vi "UI - Initiate Connection.vi"(8 "error in (no error)":errorcluster, 10 "Controller Address":string, 11 "Message Queue":refnum<queue>) -> (0 "error out":errorcluster, 1 "Connected?":bool, 3 "dup Message Queue":refnum<queue>)   [LabVIEW 2017]
uses:
  Support/Message Queue/Message Cluster.ctl
  Controls/Manual Control.ctl
  Controls/Variable References.ctl
  Globals/Host/Global - Configuration Options.vi
  Globals/Host/Global - UI Streams and Variables.vi
  Support/Message Queue/Message Queue.lvlib
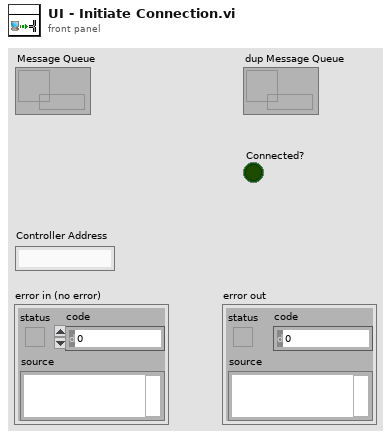
[diagram p1: front panel]
types:
  T1 = typedef "Manual Control.ctl" = cluster{"Actuator Settings":cluster{"Actuator Name":string, "Unpowered State":i16, "Output Port":u32, "Emergency State":i16, "Blank Button":bool, "Open Time [ms]":i16, "Close Time [ms]":i16}[]}
  T2 = typedef "Message Queue.lvlib/Message Cluster.ctl" = cluster{"Message":string, "Message Data":variant}
  T3 = typedef "Variable References.ctl" = cluster{"CPU Usage":refnum<k21>, "Buffer Backlog":refnum<k21>, "Contiguous Memory":refnum<k21>, "Drive Space":refnum<k21>, "Actual Loop Period":refnum<k21>, "LC Data":refnum<k21>, "PS Data":refnum<k21>, "TC Data":refnum<k21>, "Valve States":refnum<k21>, "AC Timer":refnum<k21>}
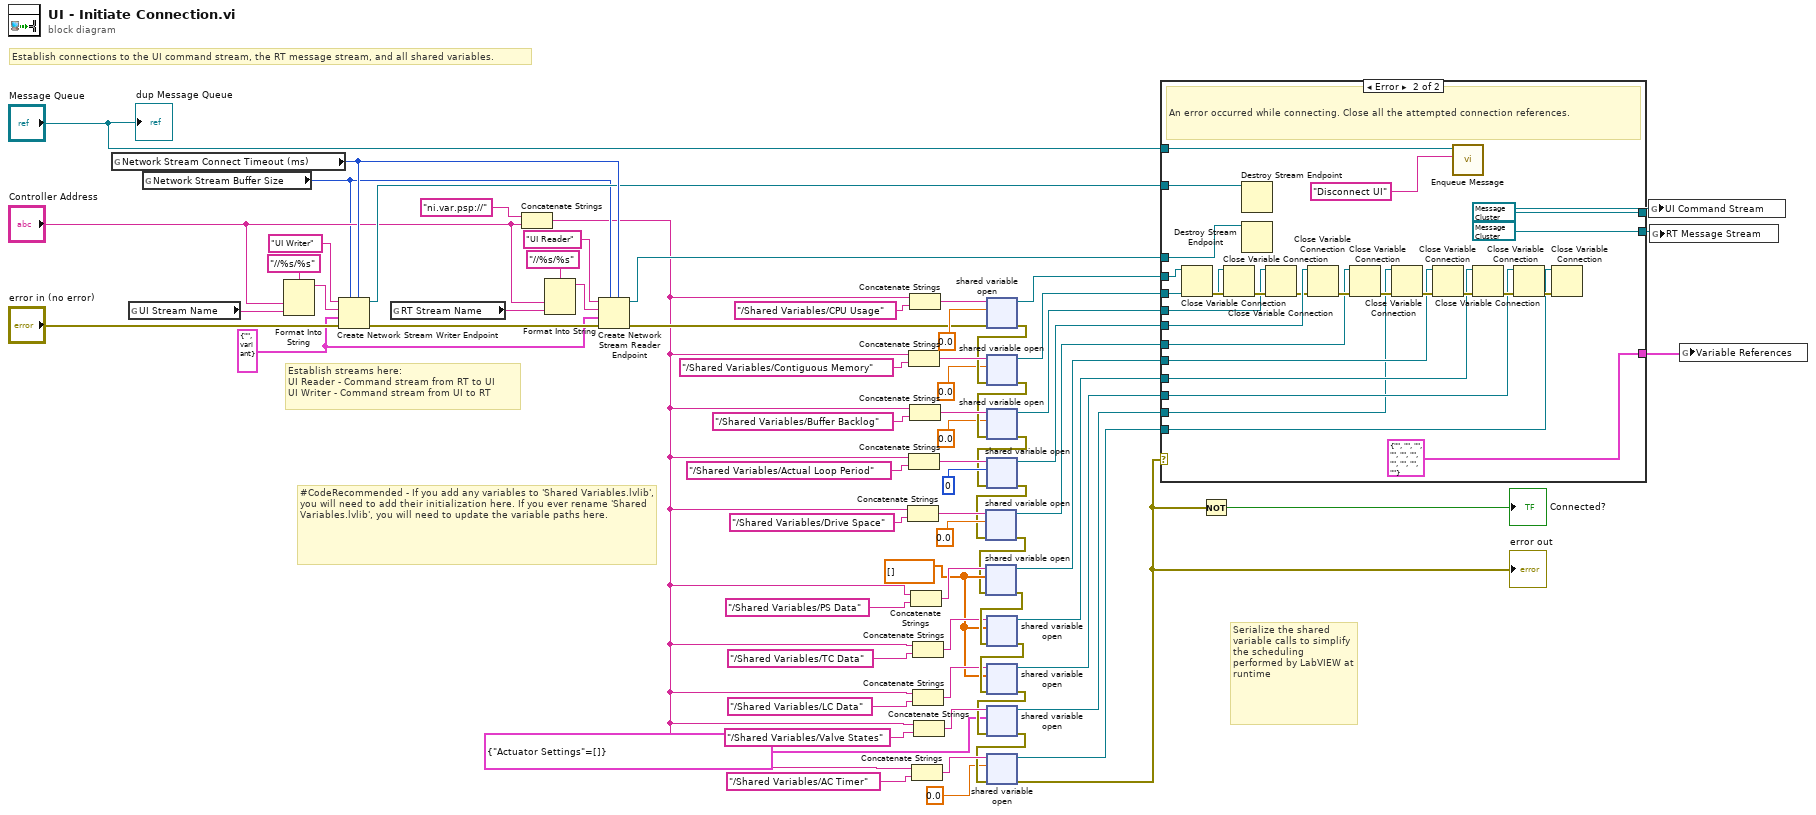
[diagram p0: block diagram]
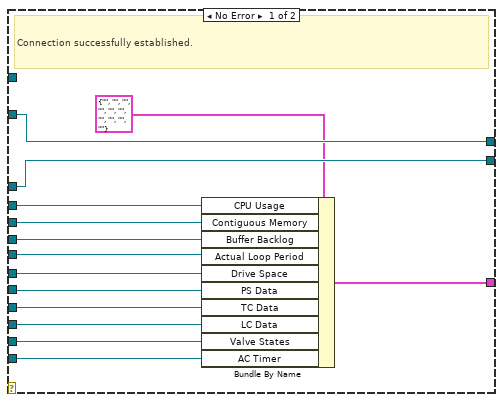
[diagram p2: hidden frame]
diagram:
  w20 = dbl[] []
  w29 = T2 {"Message"="", "Message Data"=variant} ("Message Cluster")
  # "Establish connections to the UI command stream, the RT message stream, and all shared variables."
  # "#CodeRecommended - If you add any variables to 'Shared Variables.lvlib', you will need to add their initialization here. If you ever rename 'Shared Variables.lvlib', you will need to update the variable paths here."
  # "Establish streams here:\nUI Reader - Command stream from RT to UI\nUI Writer - Command stream from UI to RT"
  # "Serialize the shared variable calls to simplify the scheduling performed by LabVIEW at runtime"
  n1 = global read "Global - Configuration Options.vi" "Network Stream Connect Timeout (ms)"() -> (w61:i32)
  n2 = global read "Global - Configuration Options.vi" "UI Stream Name"() -> (w67:string)
  n3 = global read "Global - Configuration Options.vi" "Network Stream Buffer Size"() -> (w31:i32)
  n4 = Format Into String(format string="//%s/%s", "Controller Address", w67) -> (resulting string=w66:string)  [unwired: 2 in, 1 out]
  n5 = Create Network Stream Writer Endpoint(5:w61, 7:w31, 8:"error in (no error)", 9:w29, 10:w66, 11:"UI Writer" ("reader name")) -> (0:w62:errorcluster, 3:w41:refnum<k21>)  [unwired: 1 in]
  n6 = global read "Global - Configuration Options.vi" "RT Stream Name"() -> (w70:string)
  n7 = Concatenate Strings("ni.var.psp://", "Controller Address") -> (w9:string)
  n8 = Format Into String(format string="//%s/%s", "Controller Address", w70) -> (resulting string=w69:string)  [unwired: 2 in, 1 out]
  n9 = Create Network Stream Reader Endpoint(5:w61, 7:w31, 8:w62, 9:w29, 10:w69, 11:"UI Reader" ("writer name")) -> (0:w58:errorcluster, 3:w42:refnum<k21>)  [unwired: 1 in]
  n10 = Concatenate Strings(w9, "/Shared Variables/Drive Space") -> (w36:string)
  n11 = Concatenate Strings(w9, "/Shared Variables/Contiguous Memory") -> (w54:string)
  n12 = Concatenate Strings(w9, "/Shared Variables/Actual Loop Period") -> (w50:string)
  n13 = Concatenate Strings(w9, "/Shared Variables/CPU Usage") -> (w57:string)
  n14 = Concatenate Strings(w9, "/Shared Variables/Buffer Backlog") -> (w53:string)
  n15 = Concatenate Strings(w9, "/Shared Variables/PS Data") -> (w23:string)
  n16 = Concatenate Strings(w9, "/Shared Variables/AC Timer") -> (w11:string)
  n17 = Concatenate Strings(w9, "/Shared Variables/TC Data") -> (w24:string)
  n18 = Concatenate Strings(w9, "/Shared Variables/LC Data") -> (w21:string)
  n19 = Concatenate Strings(w9, "/Shared Variables/Valve States") -> (w10:string)
  n20 = shared-variable-open(w57, w58, 0.0) -> (w46:refnum<k21>, w48:errorcluster)  [unwired: 1 in]
  n21 = shared-variable-open(w54, w48, 0.0) -> (w45:refnum<k21>, w47:errorcluster)  [unwired: 1 in]
  n22 = shared-variable-open(w53, w47, 0.0) -> (w44:refnum<k21>, w40:errorcluster)  [unwired: 1 in]
  n23 = shared-variable-open(w50, w40, u32 0) -> (w43:refnum<k21>, w35:errorcluster)  [unwired: 1 in]
  n24 = shared-variable-open(w36, w35, 0.0) -> (w34:refnum<k21>, w1:errorcluster)  [unwired: 1 in]
  n25 = shared-variable-open(w23, w1, w20) -> (w19:refnum<k21>, w25:errorcluster)  [unwired: 1 in]
  n26 = shared-variable-open(w24, w25, w20) -> (w18:refnum<k21>, w22:errorcluster)  [unwired: 1 in]
  n27 = shared-variable-open(w21, w22, w20) -> (w17:refnum<k21>, w8:errorcluster)  [unwired: 1 in]
  n28 = shared-variable-open(w10, w8, T1 {"Actuator Settings"=[]} ("Valve States")) -> (w3:refnum<k21>, w7:errorcluster)  [unwired: 1 in]
  n29 = shared-variable-open(w11, w7, 0.0) -> (w2:refnum<k21>, w6:errorcluster)  [unwired: 1 in]
  "error out" <- w6
  n30 = case shown="Error" w6 {
    tunnel: w46 -> [w82 w108]
    tunnel: w45 -> [w76 w105]
    tunnel: w44 -> [w75 w106]
    tunnel: w43 -> [w74 w107]
    tunnel: w42 -> [w84 w111]
    tunnel: w41 -> [w85 w112]
    tunnel: [w86 T3 {"CPU Usage"="", "Buffer Backlog"="", "Contiguous Memory"="", "Drive Space"="", "Actual Loop Period"="", "LC Data"="", "PS Data"="", "TC Data"="", "Valve States"="", "AC Timer"=""} ("Variable References")] -> w16
    tunnel: [w85 refnum<k21> refnum] -> w15
    tunnel: [w84 refnum<k21> refnum] -> w14
    tunnel: w34 -> [w73 w102]
    tunnel: "Message Queue" -> [_ w97]
    tunnel: w19 -> [w77 w95]
    tunnel: w18 -> [w78 w92]
    tunnel: w17 -> [w79 w91]
    tunnel: w3 -> [w80 w89]
    tunnel: w2 -> [w81 w87]
    frame No Error {
      # "Connection successfully established."
      n31 = Bundle By Name(cluster=T3 {"CPU Usage"="", "Buffer Backlog"="", "Contiguous Memory"="", "Drive Space"="", "Actual Loop Period"="", "LC Data"="", "PS Data"="", "TC Data"="", "Valve States"="", "AC Timer"=""} ("Variable References"), "CPU Usage"=w82, "Contiguous Memory"=w76, "Buffer Backlog"=w75, "Actual Loop Period"=w74, "Drive Space"=w73, "PS Data"=w77, "TC Data"=w78, "LC Data"=w79, "Valve States"=w80, "AC Timer"=w81) -> (w86:T3)
    }
    frame Error {
      # "An error occurred while connecting. Close all the attempted connection references."
      n32 = Close Variable Connection(11:w108) -> (0:w109:errorcluster)  [unwired: 1 in]
      n33 = Close Variable Connection(8:w109, 11:w105) -> (0:w110:errorcluster)
      n34 = Destroy Stream Endpoint(11:w112) -> ()  [unwired: 1 in, 1 out]
      n35 = Destroy Stream Endpoint(11:w111) -> ()  [unwired: 1 in, 1 out]
      n36 = Close Variable Connection(8:w110, 11:w106) -> (0:w104:errorcluster)
      n37 = Close Variable Connection(8:w104, 11:w107) -> (0:w103:errorcluster)
      n38 = Close Variable Connection(8:w103, 11:w102) -> (0:w101:errorcluster)
      n39 = Close Variable Connection(8:w101, 11:w89) -> (0:w100:errorcluster)
      n40 = Close Variable Connection(8:w100, 11:w95) -> (0:w94:errorcluster)
      n41 = call "Enqueue Message.vi"("Message"="Disconnect UI", "Message Queue"=w97) -> ()  [unwired: 8 in, 2 out]
      n42 = Close Variable Connection(8:w94, 11:w92) -> (0:w93:errorcluster)
      n43 = Close Variable Connection(8:w93, 11:w91) -> (0:w88:errorcluster)
      n44 = Close Variable Connection(8:w88, 11:w87) -> ()  [unwired: 1 out]
    }
  }
  n45 = Not(x=w6) -> (.not. x?=→"Connected?":bool)
  n46 = global write "Global - UI Streams and Variables.vi" "UI Command Stream"(w15) -> ()
  n47 = global write "Global - UI Streams and Variables.vi" "RT Message Stream"(w14) -> ()
  n48 = global write "Global - UI Streams and Variables.vi" "Variable References"(w16) -> ()
  "dup Message Queue" <- "Message Queue"
